vi "Compare Slaves.vi"(8 "error in (no error)":errorcluster, 11 "ECAT Slaves in":T3 {"ECAT Slave refs" format="%.0x"}) -> (0 "error out":errorcluster, 3 "ECAT Slaves out":T2(array[cluster]) {"VS ref" format="%.0x"})   [LabVIEW 2019, in "SEECD Engine.lvlib"]
uses:
  SEECD Engine.lvlib
  <vilib>/NI VeriStand/Custom Device API/Custom Device Item Ref.ctl
  Shared/Globals/Property Strings.vi
  <vilib>/NI VeriStand/Custom Device API/Get Item Property (U16).vi
  Shared/Globals/Error Strings.vi
  <vilib>/NI VeriStand/Custom Device API/Custom Device API.lvlib
  Shared/SEECD Shared.lvlib
  <resource>/objmgr/IndComECAT.rc
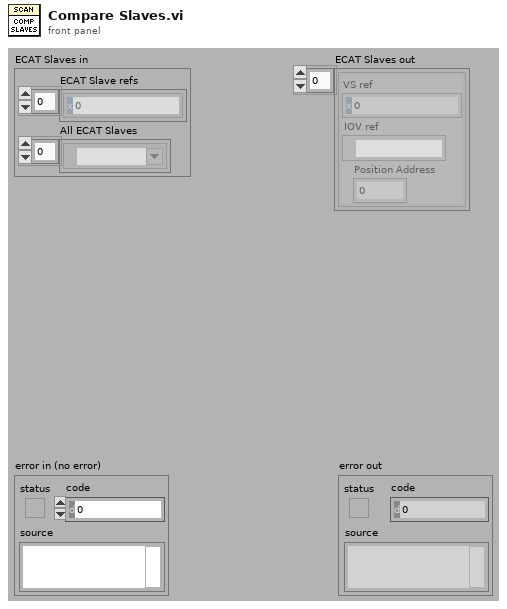
[diagram p1: front panel]
types:
  T1 = typedef "Custom Device API.lvlib/Custom Device Item Ref.ctl" = u64
  T2 = cluster{"VS ref":T1, "IOV ref":refnum<k21>, "Position Address":u16}[]
  T3 = cluster{"ECAT Slave refs":T1[], "All ECAT Slaves":refnum<k21>[]}
  T4 = cluster{"VS ref":T1, "IOV ref":refnum<k21>, "Position Address":u16}
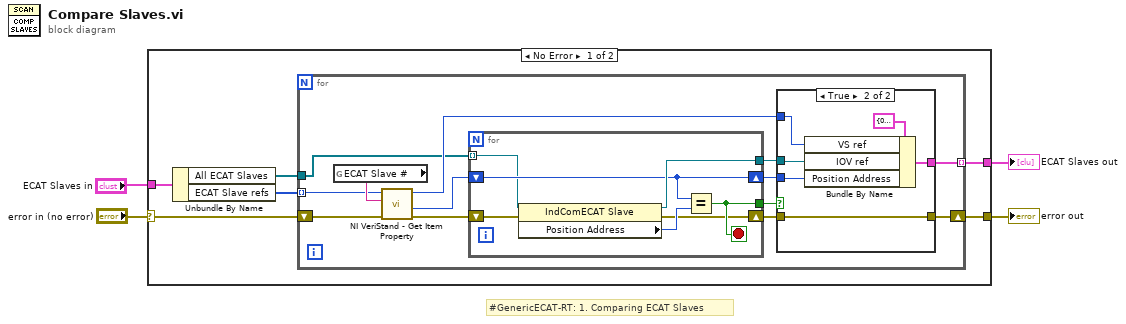
[diagram p0: block diagram]
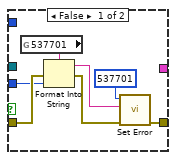
[diagram p2: hidden frame]
diagram:
  # "#GenericECAT-RT: 1. Comparing ECAT Slaves"
  n1 = case shown="No Error" "error in (no error)" {
    selector: "error in (no error)" -> [w7 w44]
    tunnel: [w6 w44] -> w3
    tunnel: "ECAT Slaves in" -> [w10 _]
    tunnel: [w5 _] -> w1
    frame No Error {
      n2 = Unbundle By Name(w10) -> ("All ECAT Slaves"=w8:refnum<k21>[], "ECAT Slave refs"=w9:T1[])
      n3 = for {
        tunnel: w9 -> [w22] mode=indexing
        tunnel: w8 -> [w12]
        shift-right: [w18] -> w6
        shift-left: w7 -> [w21]
        tunnel: [w14] -> w5 mode=indexing
        n4 = global read "Property Strings.vi" "ECAT Slave #"() -> (w23:string)
        n5 = call-poly <vilib>:"NI VeriStand - Get Item Property.vi"("error in (no error)"=w21, "Property Name"=w23, "Item Ref in"=w22) -> ("error out"=w11:errorcluster, "Value"=w13:u16, "Item Ref out"=w17:T1)  [unwired: 5 in, 1 out]
        n6 = for {
          tunnel: w12 -> [w24] mode=indexing
          shift-right: [w26] -> w19
          shift-left: w11 -> [w25]
          tunnel: [w30] -> w20
          tunnel: [w29] -> w16
          shift-right: [w27] -> w15
          shift-left: w13 -> [w27]
          stop <- w30 stop-if-true
          n7 = property class="IndComECAT Slave"(reference=w24, error in=w25) -> (reference out=w29:refnum<k21>, error out=w26:errorcluster, "Position Address"=w28:u16)
          n8 = Equal?(x=w27, y=w28) -> (x = y?=w30:bool)
        }
        n9 = case shown="True" w20 {
          tunnel: [w33 w43] -> w18
          tunnel: w19 -> [w37 w43]
          tunnel: w17 -> [_ w40]
          tunnel: w16 -> [_ w41]
          tunnel: w15 -> [w36 w42]
          tunnel: [_ w39] -> w14
          frame False {
            n10 = global read "Error Strings.vi" "537701"() -> (w32:string)
            n11 = Format Into String(format string=w32, error in=w37, w36) -> (resulting string=w35:string, error out=w34:errorcluster)  [unwired: 1 in]
            n12 = call "Set Error.vi"("error in (no error)"=w34, "Message"=w35, "Code"=537701 ("code")) -> ("error out"=w33:errorcluster)  [unwired: 8 in]
          }
          frame True {
            n13 = Bundle By Name(cluster=T4 {"VS ref"=0, "IOV ref"="", "Position Address"=0} ("EtherCAT Slave"), "VS ref"=w40, "IOV ref"=w41, "Position Address"=w42) -> (w39:T4)
          }
        }
      }
    }
    frame Error {
    }
  }
  "error out" <- w3
  "ECAT Slaves out" <- w1
